vi "setBurstPhase.vi"(7 "Burst":bool, 8 "error in (no error)":errorcluster, 10 "Phase":dbl=180.0, 11 "VISA resource name":refnum<visa-resource-name>) -> (0 "error out":errorcluster, 3 "VISA resource name out":refnum<visa-resource-name>)   [LabVIEW 2023, in "Keysight-33500B.lvlib"]
doc: "<b>Author:</b> Wolfgang\n<b>Description:</b>\nSets the starting phase angle for the burst. in degree"
uses:
  Keysight-33500B.lvlib
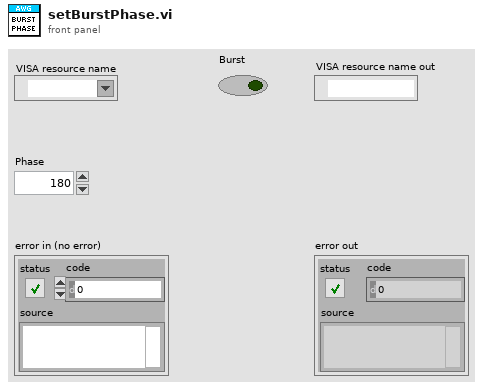
[diagram p1: front panel]
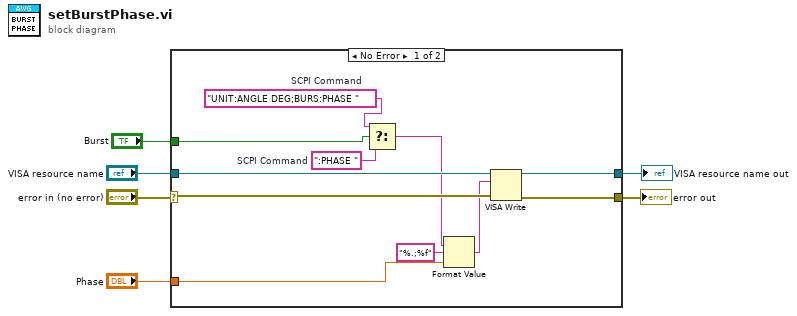
[diagram p0: block diagram]
diagram:
  n1 = case shown="No Error" "error in (no error)" {
    selector: "error in (no error)" -> [w14 w19]
    tunnel: [w16 w18] -> w6
    tunnel: [w17 w19] -> w4
    tunnel: "VISA resource name" -> [w15 w18]
    tunnel: "Phase" -> [w13 _]
    tunnel: "Burst" -> [w10 _]
    frame No Error {
      w7 = ":PHASE "  # SCPI Command
      w9 = "UNIT:ANGLE DEG;BURS:PHASE "  # SCPI Command
      n2 = Select(t=w9, s=w10, f=w7) -> (s? t:f=w8:string)
      n3 = Format Value(string ("")=w8, format string="%.;%f", value (0)=w13) -> (output string=w12:string)
      n4 = VISA Write(VISA resource name=w15, write buffer=w12, error in (no error)=w14) -> (VISA resource name out=w16:refnum<visa-resource-name>, error out=w17:errorcluster)  [unwired: 1 out]
    }
    frame Error {
    }
  }
  "VISA resource name out" <- w6
  "error out" <- w4
